vi "Read Enc.vi"(8 "error in (no error)":errorcluster, 10 "Reset Counter":bool, 11 "SGDV_Ctrl_Class in":refnum<class "SGDV_Ctrl_Class.lvclass">) -> (0 "error out":errorcluster, 2 "Pos Passed(deg)":dbl, 3 "SGDV_Ctrl_Class out":refnum<class "SGDV_Ctrl_Class.lvclass">)   [LabVIEW 2013, in "SGDV_Ctrl_v13_lib.lvlib" / "SGDV_Ctrl_Class.lvclass"]
uses:
  SGDV_Ctrl_Class.lvclass
  SGDV_Ctrl_Class.lvclass/SGDV_Ctrl_Class.ctl
  SGDV_Ctrl_v13_lib.lvlib
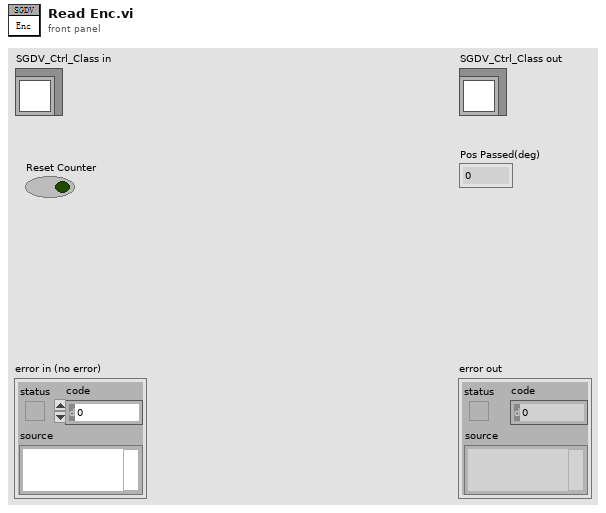
[diagram p1: front panel]
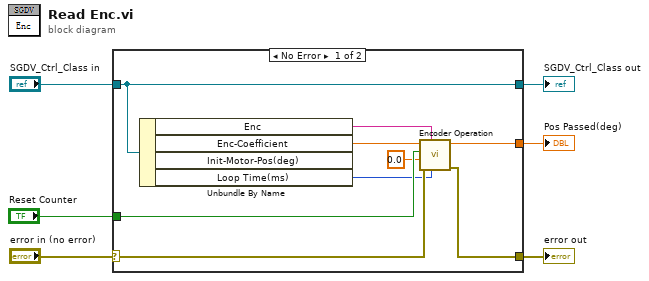
[diagram p0: block diagram]
diagram:
  n1 = case shown="No Error" "error in (no error)" {
    selector: "error in (no error)" -> [w12 w16]
    tunnel: [w11 w16] -> w5
    tunnel: [w15 w17] -> w3
    tunnel: "SGDV_Ctrl_Class in" -> [w15 w17]
    tunnel: "Reset Counter" -> [w13 _]
    tunnel: [w7 _] -> w1
    frame No Error {
      n2 = Unbundle By Name(w15) -> ("Enc"=w14:tag, "Enc-Coefficient"=w9:dbl, "Loop Time(ms)"=w10:u32)  [unwired: 1 out]
      n3 = call "Encoder Operation.vi"("Loop Time(ms)"=w10, "Enc"=w14, "error in (no error)"=w12, "Init-Enc-Pos"=0.0, "Reset Counter"=w13, "Enc-Coefficient"=w9) -> ("error out"=w11:errorcluster, "Pos Passed(deg)"=w7:dbl)  [unwired: 1 in, 3 out]
    }
    frame Error {
    }
  }
  "error out" <- w5
  "SGDV_Ctrl_Class out" <- w3
  "Pos Passed(deg)" <- w1
